vi "Exercise4.6-FM_RTL-SDR_RX - FIR--V2.vi"() -> ()   [LabVIEW 2013]
uses:
  <vilib>/sound2/lvsound2.llb/Sound Data Format.ctl
  <vilib>/sound2/lvsound2.llb/Sound Output Write (DBL Single).vi
  <instrlib>/rtlsdr/rtlsdr.lvlib
panel:
  out "FM Spectrum":cluster{dbl[], dbl[]}[](graph)
  out "Boolean":bool
  in  "Device index":u32
  out "Samples Acquired":u32
  out "# elements in queue":i32
  out "DevRefnum":u64
  out "XY Graph":cluster{dbl[], dbl[]}(graph)
  out "error out":errorcluster
  in  "sound format":T1={"sample rate (S/s)"=44100.0, "number of channels"=1, "bits per sample"=16}
  in  "stop":bool
  in  "Center frequency":u32=92700000
  in  "IQ rate":u32=286650
  out "error out":errorcluster
  # "FM Receiver"
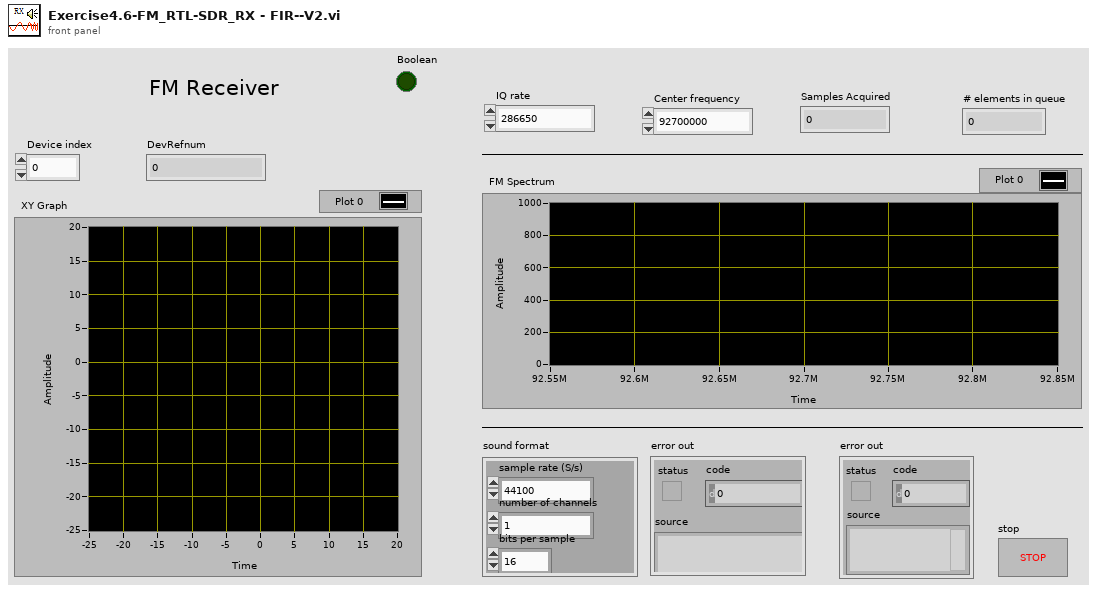
[diagram p1: front panel]
types:
  T1 = typedef "Sound Data Format.ctl" = cluster{"sample rate (S/s)":dbl, "number of channels":i32, "bits per sample":i32}
  T2 = typedef "Sound Output Task ID.ctl" = u32
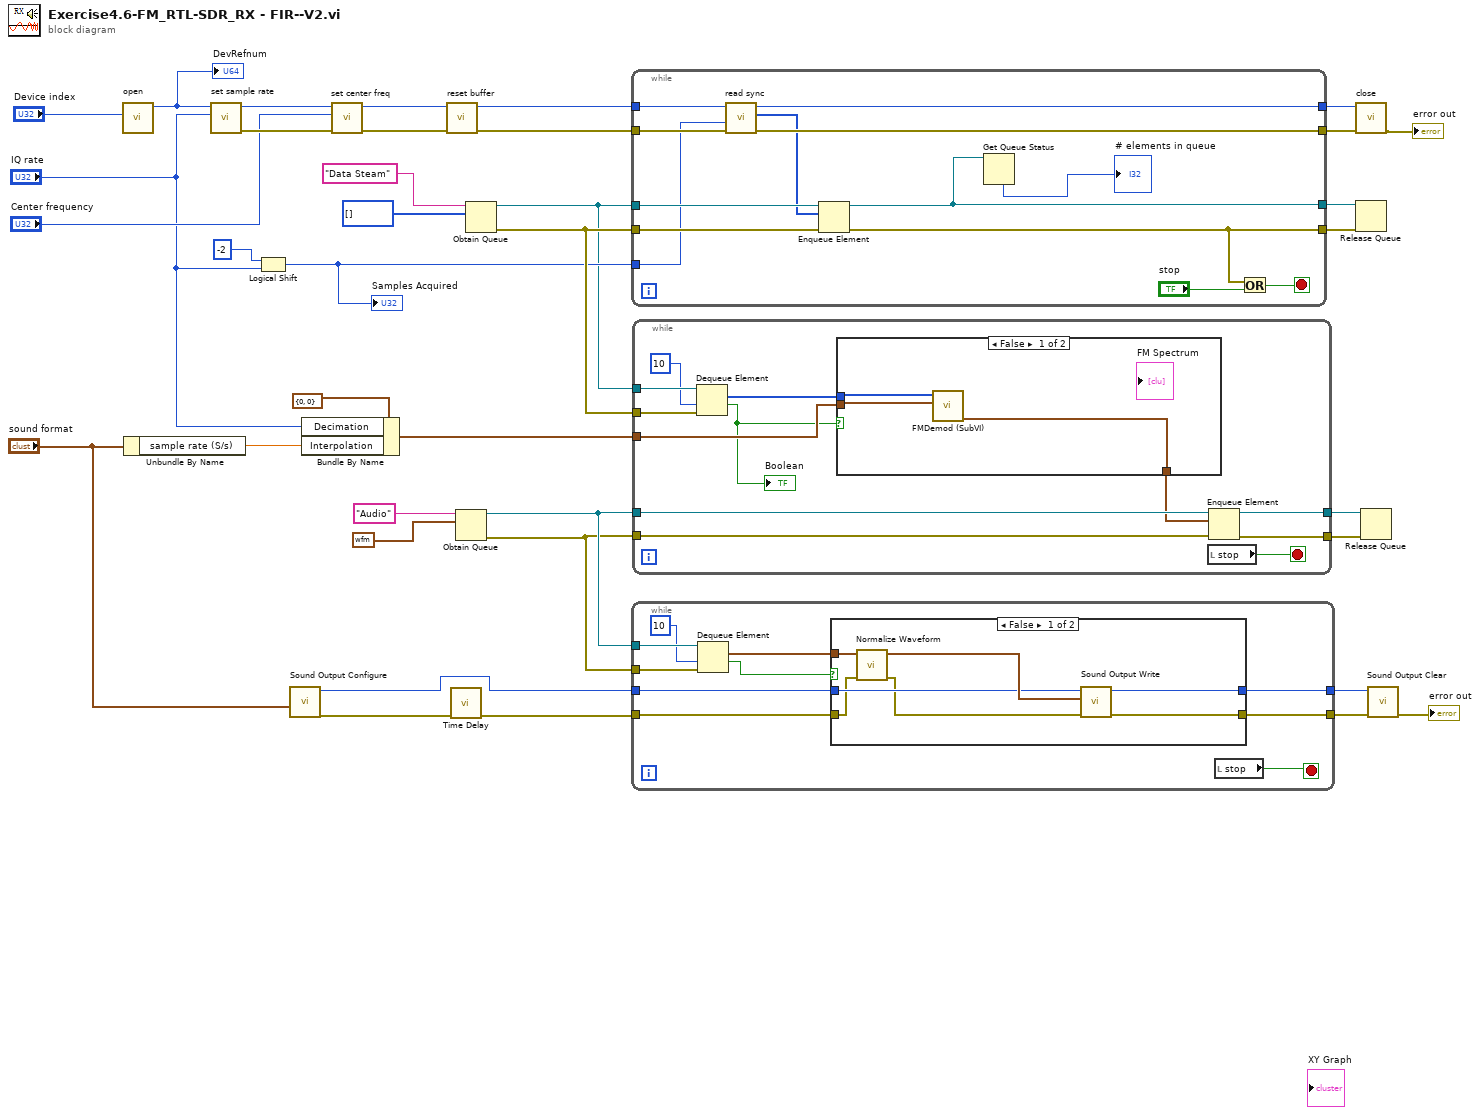
[diagram p0: block diagram]
diagram:
  n1 = call <instrlib>:"open.vi"("index"="Device index") -> ("DevRefnum"=w30:u64)  [unwired: 9 in, 1 out]
  "DevRefnum" <- w30
  n2 = Unbundle By Name("sound format") -> ("sample rate (S/s)"=w23:dbl)
  n3 = call <instrlib>:"set sample rate.vi"("rate"="IQ rate", "DevRefnum"=w30) -> ("error out"=w32:errorcluster, "DevRefnum"=w34:u64)  [unwired: 7 in, 1 out]
  n4 = Logical Shift(y=i16 -2, x="IQ rate") -> (x << y=w15:u32)
  "Samples Acquired" <- w15
  n5 = call <vilib>:"Sound Output Configure.vi"("sound format"="sound format") -> ("error out"=w5:errorcluster, "task ID"=w3:T2)  [unwired: 9 in]
  n6 = Bundle By Name(cluster=cluster{"Interpolation":i32, "Decimation":i32} {"Interpolation"=0, "Decimation"=0}, "Decimation"="IQ rate", "Interpolation"=w23) -> (w18:cluster{"Interpolation":i32, "Decimation":i32})
  n7 = call <instrlib>:"set center freq.vi"("error in (no error)"=w32, "freq"="Center frequency", "DevRefnum"=w34) -> ("error out"=w31:errorcluster, "DevRefnum"=w33:u64)  [unwired: 6 in, 1 out]
  n8 = call <instrlib>:"reset buffer.vi"("error in (no error)"=w31, "DevRefnum"=w33) -> ("error out"=w28:errorcluster, "DevRefnum"=w29:u64)  [unwired: 8 in]
  n9 = call "Time Delay"("error in (no error)"=w5) -> ("error out"=w4:errorcluster)  [unwired: 10 in]
  n10 = Obtain Queue(name (unnamed)="Audio", element data type=waveform(dbl) {"t0"=timestamp(0 s since 1904-01-01), "dt"=1.0, "Y"=[]} ("Waveform")) -> (queue out=w10:refnum<queue>, error out=w9:errorcluster)  [unwired: 3 in, 1 out]
  n11 = Obtain Queue(name (unnamed)="Data Steam", element data type=u8[] [] ("buf 2")) -> (queue out=w14:refnum<queue>, error out=w16:errorcluster)  [unwired: 3 in, 1 out]
  n12 = while {
    tunnel: [w48] -> w26
    tunnel: w29 -> [w50]
    tunnel: w28 -> [w49]
    tunnel: [w47] -> w25
    tunnel: w15 -> [w38]
    tunnel: w14 -> [w45]
    tunnel: [w44] -> w21
    tunnel: w16 -> [w43]
    tunnel: [w41] -> w20
    stop <- w39 stop-if-true
    n13 = call <instrlib>:"read sync.vi"("error in (no error)"=w49, "len"=w38, "DevRefnum"=w50) -> ("error out"=w47:errorcluster, "buf 2"=w42:u8[], "DevRefnum"=w48:u64)  [unwired: 6 in]
    n14 = Enqueue Element(queue=w45, element=w42, error in (no error)=w43) -> (queue out=w44:refnum<queue>, error out=w41:errorcluster)  [unwired: 1 in, 1 out]
    n15 = Get Queue Status(queue=w44) -> (# elements in queue=→"# elements in queue":i32)  [unwired: 2 in, 7 out]
    n16 = Or(x=w41, y="stop") -> (x .or. y?=w39:bool)
  }
  n17 = while {
    tunnel: w10 -> [w60]
    tunnel: w9 -> [w59]
    tunnel: w4 -> [w58]
    tunnel: [w57] -> w8
    tunnel: w3 -> [w55]
    tunnel: [w54] -> w7
    stop <- w52 stop-if-true
    n18 = Dequeue Element(queue=w60, timeout in ms (-1)=10, error in (no error)=w59) -> (element=w56:waveform(dbl), timed out?=w53:bool)  [unwired: 2 out]
    n19 = case shown="False" w53 {
      tunnel: w58 -> [w62 w68]
      tunnel: [w63 w68] -> w57
      tunnel: w56 -> [w66 _]
      tunnel: w55 -> [w65 w69]
      tunnel: [w64 w69] -> w54
      frame False {
        n20 = call <vilib>:"Normalize Waveform.vi"("error in (no error)"=w62, "waveform in"=w66) -> ("error out"=w61:errorcluster, "normalized waveform"=w67:waveform(dbl))  [unwired: 6 in, 2 out]
        n21 = call-poly <vilib>:"Sound Output Write.vi"("error in (no error)"=w61, "data"=w67, "task ID"=w65) -> ("error out"=w63:errorcluster, "task ID out"=w64:T2)  [unwired: 7 in]
      }
      frame True {
      }
    }
    n22 = local read "stop"() -> (w52:bool)
  }
  n23 = while {
    tunnel: w14 -> [w81]
    tunnel: w18 -> [w78]
    tunnel: w16 -> [w79]
    tunnel: w10 -> [w77]
    tunnel: [w76] -> w12
    tunnel: [w75] -> w11
    tunnel: w9 -> [w74]
    stop <- w71 stop-if-true
    n24 = Dequeue Element(queue=w81, timeout in ms (-1)=10, error in (no error)=w79) -> (element=w80:u8[], timed out?=w70:bool)  [unwired: 2 out]
    "Boolean" <- w70
    n25 = case shown="False" w70 {
      tunnel: w80 -> [w84 _]
      tunnel: w78 -> [w83 _]
      tunnel: [w82 _] -> w73
      frame False {
        n26 = call "FMDemod (SubVI).vi"("Cluster"=w83, "buf in"=w84) -> ("Waveform"=w82:waveform(dbl))  [unwired: 8 in, 1 out]
      }
      frame True {
      }
    }
    n27 = local read "stop"() -> (w71:bool)
    n28 = Enqueue Element(queue=w77, element=w73, error in (no error)=w74) -> (queue out=w76:refnum<queue>, error out=w75:errorcluster)  [unwired: 1 in, 1 out]
  }
  n29 = call <instrlib>:"close.vi"("error in (no error)"=w25, "DevRefnum"=w26) -> ("error out"=→"error out":errorcluster)  [unwired: 8 in, 1 out]
  n30 = Release Queue(queue=w21, error in (no error)=w20) -> ()  [unwired: 1 in, 3 out]
  n31 = Release Queue(queue=w12, error in (no error)=w11) -> ()  [unwired: 1 in, 3 out]
  n32 = call <vilib>:"Sound Output Clear.vi"("error in (no error)"=w8, "task ID"=w7) -> ("error out"=→"error out":errorcluster)  [unwired: 9 in]
